vi "FIR Filter for 1 Chan (CDB).vi"(4 "optional FIR filter specifications":T2={"PB Gain"=-3.0, "SB Gain"=-60.0, "Scale"=TRUE, "Window"=enum."Flat Top"} {"SB Gain" format="%.2p"; "PB Gain" format="%.2p"}, 6 "FIR filter specifications":T3={"Topology"=enum."Off", "Type"=enum."Lowpass", "#Taps"=50, "Lower PB"=100.0, "Upper PB"=0.0, "Lower SB"=200.0, "Upper SB"=0.0} {"Lower SB" format="%0.2p"; "Upper SB" format="%0.2p"; "Lower PB" format="%0.2p"; "Upper PB" format="%0.2p"}, 7 "reset filter":bool, 8 "error in (no error)":errorcluster, 11 "signal in":waveform(cdb)={"t0"=timestamp(0 s since 1904-01-01), "dt"=0.001, "Y"=[]}) -> (0 "error out":errorcluster, 2 "filter information":T1 {"phase H(w)"."df" format="%.2p"; "phase H(w)"."f0" format="%.2p"; "phase H(w)"."Phase H(w)" format="%.2p"; "magnitude H(w)"."df" format="%.2p"; "magnitude H(w)"."f0" format="%.2p"; "magnitude H(w)"."Mag H(w)" format="%.2p"}, 3 "signal out":waveform(cdb))   [LabVIEW 2020, in "NI_MAPro.lvlib"]
doc: "Filters signals in either single or multiple waveforms. If you are filtering multiple waveforms, the VI maintains separate filter states for each waveform. The data types you wire to the <B>signal in</B> and <B>FIR filter specifications</B> inputs determine the polymorphic instance to use."
uses:
  NI_MAPro.lvlib
  NI_MABase.lvlib
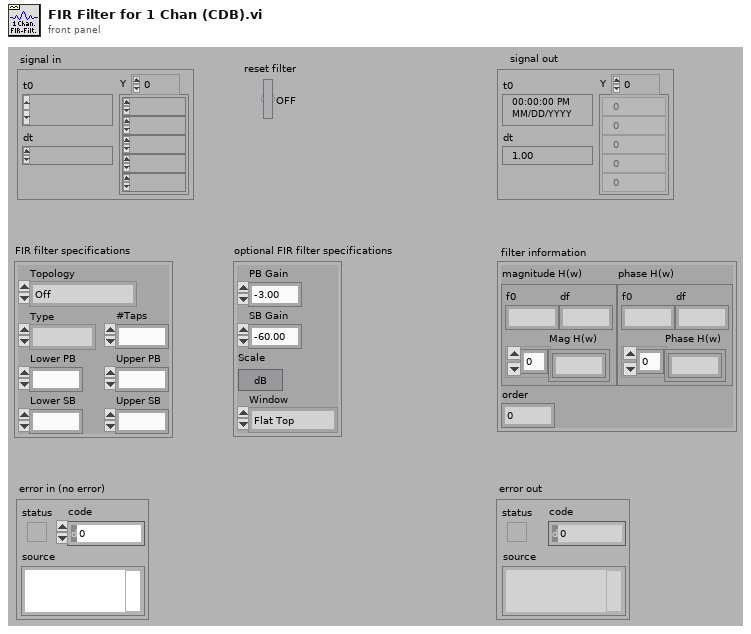
[diagram p1: front panel]
types:
  T1 = cluster{"magnitude H(w)":cluster{"f0":dbl, "df":dbl, "Mag H(w)":dbl[]}, "phase H(w)":cluster{"f0":dbl, "df":dbl, "Phase H(w)":dbl[]}, "order":i32}
  T2 = cluster{"PB Gain":dbl, "SB Gain":dbl, "Scale":bool, "Window":enum16{"None", "Hanning", "Hamming", "Triangular", "Blackman", "Exact Blackman", "Blackman-Harris", "Kaiser-Bessel", "Flat Top"}}
  T3 = cluster{"Topology":enum16{"Off", "FIR by Specification", "Equi-ripple FIR", "Windowed FIR"}, "Type":enum16{"Lowpass", "Highpass", "Bandpass", "Bandstop"}, "#Taps":i32, "Lower PB":dbl, "Upper PB":dbl, "Lower SB":dbl, "Upper SB":dbl}
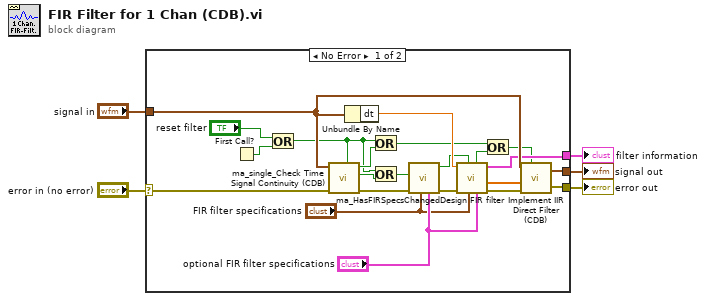
[diagram p0: block diagram]
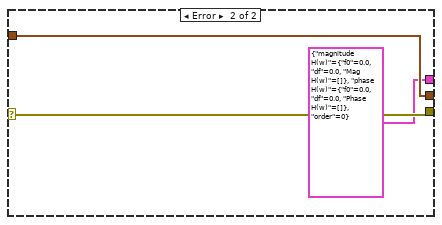
[diagram p2: hidden frame]
diagram:
  n1 = case shown="No Error" "error in (no error)" {
    selector: "error in (no error)" -> [w24 w29]
    tunnel: "signal in" -> [w25 w30]
    tunnel: [w27 w29] -> w4
    tunnel: [w26 w30] -> w3
    tunnel: [w23 T1 {"magnitude H(w)"={"f0"=0.0, "df"=0.0, "Mag H(w)"=[]}, "phase H(w)"={"f0"=0.0, "df"=0.0, "Phase H(w)"=[]}, "order"=0} ("filter information")] -> w1
    frame No Error {
      n2 = First Call?() -> (First Call?: T/F=w8:bool)
      n3 = Or(x="reset filter", y=w8) -> (x .or. y?=w6:bool)
      n4 = call "ma_single_Check Time Signal Continuity (CDB).vi"("Ignore input time stamp"=w6, "error in (no error)"=w24, "Waveform"=w25) -> ("error out"=w16:errorcluster, "dt changed"=w11:bool, "t0 changed"=w13:bool)  [unwired: 5 in, 1 out]
      n5 = Unbundle By Name(w25) -> ("dt"=w22:dbl)
      n6 = Or(x=w6, y=w13) -> (x .or. y?=w14:bool)
      n7 = Or(x=w6, y=w11) -> (x .or. y?=w12:bool)
      n8 = call "ma_HasFIRSpecsChanged.vi"("optional FIR filter specifications"="optional FIR filter specifications", "FIR Filter Specifications"="FIR filter specifications", "error in (no error)"=w16, "redesign filter"=w12) -> ("error out"=w17:errorcluster, "ValsDifferent?"=w15:bool)  [unwired: 6 in]
      n9 = call "Design FIR filter.vi"("optional FIR filter specifications"="optional FIR filter specifications", "FIR filter specifications"="FIR filter specifications", "redesign filter"=w15, "error in"=w17, "dt"=w22) -> ("error out"=w20:errorcluster, "forward coefficients"=w21:dbl[], "filter information"=w23:T1, "reset filter state"=w19:bool)  [unwired: 3 in]
      n10 = Or(x=w14, y=w19) -> (x .or. y?=w18:bool)
      n11 = call "Implement IIR Direct Filter (CDB).vi"("signal in"=w25, "forward coefficients"=w21, "error in (no error)"=w20, "reset filter"=w18) -> ("signal out"=w26:waveform(cdb), "error out"=w27:errorcluster)  [unwired: 1 in]
    }
    frame Error {
    }
  }
  "error out" <- w4
  "signal out" <- w3
  "filter information" <- w1
